vi "Compressor.vi"(8 "Mode":enum16{"Init", "Run", "End"}(ring), 9 "Compressor State":enum32{"Start", "Stop"}(radio), 10 "Digital Module A":T1={"DIO Module"=enum."Digital Module 1", "Left Encoder B Channel"=enum."DIO 1", "Left Encoder A Channel"=enum."DIO 2", "Right Encoder B Channel"=enum."DIO 3", "Right Encoder A Channel"=enum."DIO 4", "Arm Encoder A Channel"=enum."DIO 5", "Arm Encoder B Channel"=enum."DIO 6", "Pressure Switch"=enum."DIO 7", "Unassigned"=enum."DIO 8", "Unassigned"=enum."DIO 9", "Ultrasonic Trigger"=enum."DIO 10", "Remus Switch"=enum."DIO 11", "Unassigned"=enum."DIO 12", "Unassigned"=enum."DIO 13", "Unassigned"=enum."DIO 14"}, 11 "PWM Module (DIO A)":T4={"PWM Module"=enum."Digital Module 1", "Unassigned"=enum."PWM 1", "Unassigned"=enum."PWM 2", "Right Motor"=enum."PWM 3", "Left Motor"=enum."PWM 4", "Unassigned"=enum."PWM 5", "Unassigned"=enum."PWM 6", "Unassigned"=enum."PWM 7", "Arm Motor"=enum."PWM 8", "Unassigned"=enum."PWM 9", "Unassigned"=enum."PWM 10", "Compressor"=enum."Relay 1", "Unassigned"=enum."Relay 2", "Unassigned"=enum."Relay 3", "Unassigned"=enum."Relay 4", "Unassigned"=enum."Relay 5", "Unassigned"=enum."Relay 6", "Unassigned"=enum."Relay 7", "Unassigned "=enum."Relay 8"}) -> ()   [LabVIEW 2013]
doc: "Run the Compressor"
uses:
  Type Defs/PWM Module (DIO A).ctl
  <vilib>/Rock Robotics/SystemInterfaces/Typedef/FPGA_TypedefDigitalModule.ctl
  <vilib>/Rock Robotics/SystemInterfaces/DIO/FPGA_DIOPWMChannel.ctl
  <vilib>/Rock Robotics/SystemInterfaces/DIO/FPGA_DIORelayChannel.ctl
  Type Defs/Digital Module A.ctl
  <vilib>/Rock Robotics/SystemInterfaces/DIO/FPGA_DIOChannel.ctl
  <vilib>/Rock Robotics/WPI/Compressor/WPI_CompressorGetSetRefNum.vi
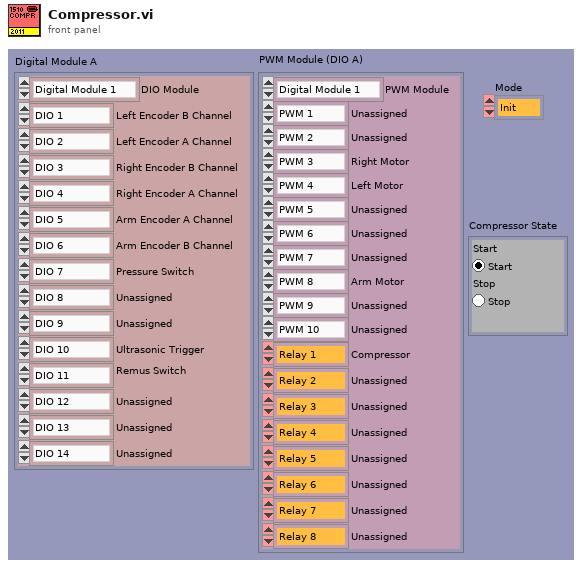
[diagram p1: front panel]
types:
  T1 = typedef "Digital Module A.ctl" = cluster{"DIO Module":T2, "Left Encoder B Channel":T3, "Left Encoder A Channel":T3, "Right Encoder B Channel":T3, "Right Encoder A Channel":T3, "Arm Encoder A Channel":T3, "Arm Encoder B Channel":T3, "Pressure Switch":T3, "Unassigned":T3, "Unassigned":T3, "Ultrasonic Trigger":T3, "Remus Switch":T3, "Unassigned":T3, "Unassigned":T3, "Unassigned":T3}
  T2 = typedef "FPGA_TypedefDigitalModule.ctl" = enum16{"Digital Module 1", "Digital Module 2"}
  T3 = typedef "FPGA_DIOChannel.ctl" = enum8{"DIO 1", "DIO 2", "DIO 3", "DIO 4", "DIO 5", "DIO 6", "DIO 7", "DIO 8", "DIO 9", "DIO 10", "DIO 11", "DIO 12", "DIO 13", "DIO 14", "Invalid"}
  T4 = typedef "PWM Module (DIO A).ctl" = cluster{"PWM Module":T2, "Unassigned":T5, "Unassigned":T5, "Right Motor":T5, "Left Motor":T5, "Unassigned":T5, "Unassigned":T5, "Unassigned":T5, "Arm Motor":T5, "Unassigned":T5, "Unassigned":T5, "Compressor":T6, "Unassigned":T6, "Unassigned":T6, "Unassigned":T6, "Unassigned":T6, "Unassigned":T6, "Unassigned":T6, "Unassigned ":T6}
  T5 = typedef "FPGA_DIOPWMChannel.ctl" = enum8{"PWM 1", "PWM 2", "PWM 3", "PWM 4", "PWM 5", "PWM 6", "PWM 7", "PWM 8", "PWM 9", "PWM 10", "Invalid"}
  T6 = typedef "FPGA_DIORelayChannel.ctl" = enum8{"Relay 1", "Relay 2", "Relay 3", "Relay 4", "Relay 5", "Relay 6", "Relay 7", "Relay 8", "Invalid"}
  T7 = typedef "WPI_CompressorDevRef.ctl" = cluster{"DevStatus":errorcluster, "DigitalInputDevRef":T8, "RelayDevRef":T9}
  T8 = typedef "WPI_DigitalInputDevRef.ctl" = cluster{"DevStatus":errorcluster, "DIO Channel":T3, "Digital Module":T2}
  T9 = typedef "WPI_RelayDevRef.ctl" = cluster{"DevStatus":errorcluster, "Relay Channel":T6, "Digital Module":T2, "Relay Direction":T10}
  T10 = typedef "WPI_RelayDirection.ctl" = enum16{"Both directions", "Forward only", "Reverse only"}
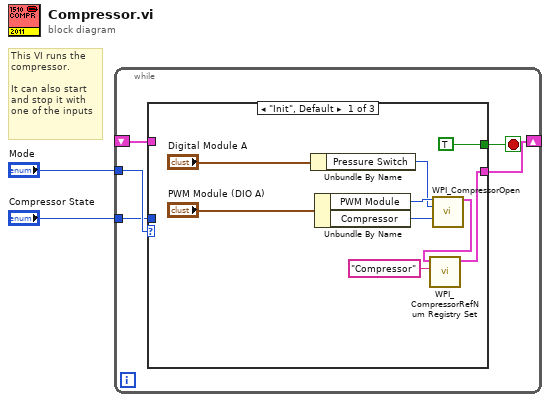
[diagram p0: block diagram]
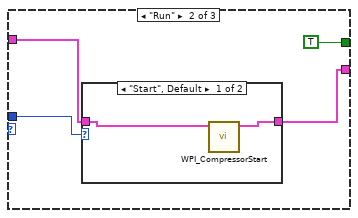
[diagram p2: hidden frame]
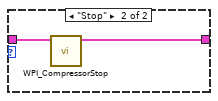
[diagram p3: hidden frame]
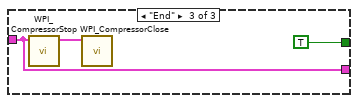
[diagram p4: hidden frame]
diagram:
  # "This VI runs the\ncompressor.\n\nIt can also start\nand stop it with\none of the inputs"
  n1 = while {
    tunnel: "Mode" -> [w7]
    shift-right: [w6] -> _
    shift-left: _ -> [w5]
    tunnel: "Compressor State" -> [w3]
    stop <- w4 stop-if-true
    n2 = case shown="\"Init\", Default" w7 {
      tunnel: [w8 w18 w26] -> w6
      tunnel: w5 -> [_ w17 w26]
      tunnel: [TRUE TRUE TRUE] -> w4
      tunnel: w3 -> [_ w19 _]
      frame "Init", Default {
        n3 = Unbundle By Name("Digital Module A") -> ("Pressure Switch"=w12:T3)
        n4 = Unbundle By Name("PWM Module (DIO A)") -> ("PWM Module"=w15:T2, "Compressor"=w14:T6)
        n5 = call <vilib>:"WPI_CompressorOpen.vi"("Pressure Switch Digital Module (Module 1)"=w15, "Pressure Switch DIO Channel"=w12, "Relay Channel"=w14) -> ("CompressorDevRef"=w10:T7)  [unwired: 2 in, 10 out]
        n6 = call <vilib>:"WPI_CompressorRefNum Registry Set.vi"("refnum name"="Compressor", "CompressorDevRef"=w10) -> ("CompressorDevRef"=w8:T7)  [unwired: 8 in, 1 out]
      }
      frame "Run" {
        n7 = case shown="\"Start\", Default" w19 {
          tunnel: w17 -> [w21 w24]
          tunnel: [w22 w23] -> w18
          frame "Start", Default {
            n8 = call <vilib>:"WPI_CompressorStart.vi"("CompressorDevRef"=w21) -> ("CompressorDevRef"=w22:T7)  [unwired: 1 in, 9 out]
          }
          frame "Stop" {
            n9 = call <vilib>:"WPI_CompressorStop.vi"("CompressorDevRef"=w24) -> ("CompressorDevRef"=w23:T7)  [unwired: 1 in, 9 out]
          }
        }
      }
      frame "End" {
        n10 = call <vilib>:"WPI_CompressorStop.vi"("CompressorDevRef"=w26) -> ("CompressorDevRef"=w27:T7)  [unwired: 1 in, 9 out]
        n11 = call <vilib>:"WPI_CompressorClose.vi"("CompressorDevRef"=w27) -> ()  [unwired: 1 in, 10 out]
      }
    }
  }
